vi "GetDataDAC.vi"(10 "data":string) -> (1 "blue":dbl, 3 "red":dbl)   [LabVIEW 2012]
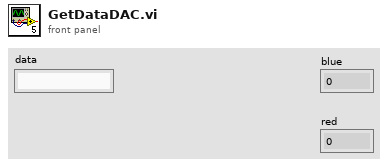
[diagram p1: front panel]
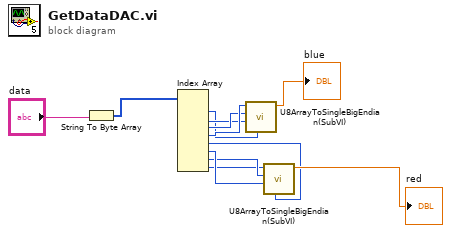
[diagram p0: block diagram]
diagram:
  n1 = String To Byte Array(string="data") -> (unsigned byte array=w2:u8[])
  n2 = Index Array(array=w2) -> (element #1=w3:u8, element #2=w4:u8, element #3=w5:u8, element #4=w6:u8, element #5=w11:u8, element #6=w10:u8, element #7=w9:u8, element #8=w8:u8)  [unwired: 8 in]
  n3 = call "U8ArrayToSingleBigEndian(SubVI).vi"("Numeric 5"=w3, "Numeric 4"=w4, "Numeric 3"=w5, "Numeric in"=w6) -> ("Numeric 8"=→"blue":sgl)  [unwired: 7 in]
  n4 = call "U8ArrayToSingleBigEndian(SubVI).vi"("Numeric 5"=w11, "Numeric 4"=w10, "Numeric 3"=w9, "Numeric in"=w8) -> ("Numeric 8"=→"red":sgl)  [unwired: 7 in]
